vi "3654SendLog.vi"() -> ()   [LabVIEW 2017]
uses:
  <vilib>/Rock Robotics/Network Tables/NT Write Numeric Array.vi
panel:
  in  "Logging":bool
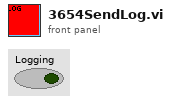
[diagram p1: front panel]
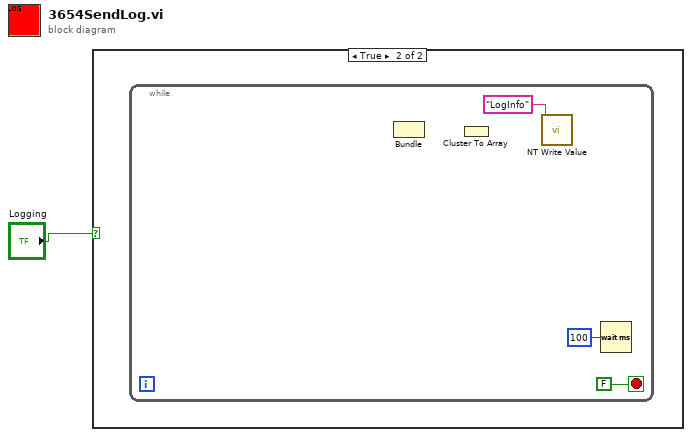
[diagram p0: block diagram]
diagram:
  n1 = case shown="True" "Logging" {
    frame False {
    }
    frame True {
      n2 = while {
        stop <- FALSE stop-if-true
        n3 = Bundle() -> ()  [unwired: 3 in, 1 out]
        n4 = Cluster To Array() -> ()  [unwired: 1 in, 1 out]
        n5 = call-poly <vilib>:"NT Write Value.vi"("Name"="LogInfo") -> ()  [unwired: 10 in, 1 out]
        n6 = Wait (ms)(milliseconds to wait=u32 100) -> ()  [unwired: 1 out]
      }
    }
  }
